vi "Data Retrim.vi"(11 "Data in":dbl[][][](array[numeric])) -> (3 "Data Out":dbl[][][](array[numeric]))   [LabVIEW 2011]
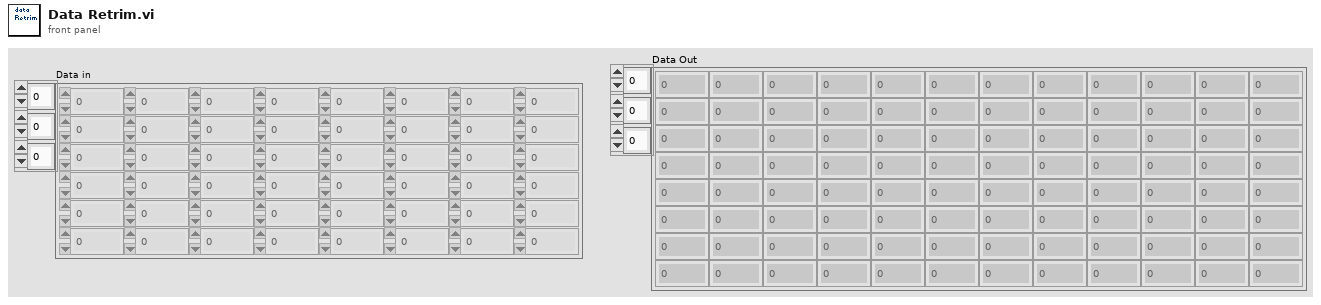
[diagram p1: front panel]
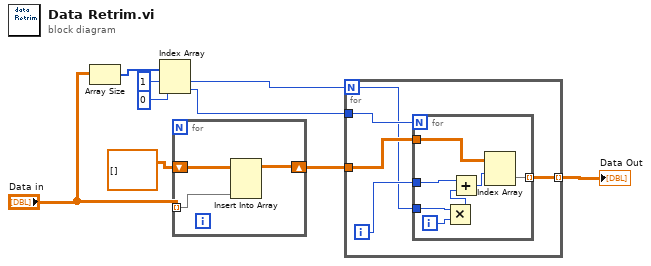
[diagram p0: block diagram]
diagram:
  n1 = Array Size(array="Data in") -> (size(s)=w6:i32[])
  n2 = Index Array(array=w6, index #1=1 ("索引"), index #2=0 ("索引")) -> (element #1=w4:i32, element #2=w2:i32)
  n3 = for {
    tunnel: "Data in" -> [w11] mode=indexing
    shift-right: [w10] -> w8
    shift-left: dbl[][] [] ("Data Out 3") -> [w12]
    n4 = Insert Into Array(array=w12, new element=w11) -> (w10:dbl[][])  [unwired: 2 in]
  }
  n5 = for {
    N: w4 -> [w13]
    tunnel: w8 -> [w17]
    tunnel: w2 -> [w16]
    tunnel: [w14] -> w1 mode=indexing
    i -> [w15]
    n6 = for {
      N: w16 -> [_]
      tunnel: w17 -> [w24]
      tunnel: w15 -> [w22]
      tunnel: [w23] -> w14 mode=indexing
      tunnel: w13 -> [w19]
      i -> [w21]
      n7 = Multiply(x=w19, y=w21) -> (x*y=w20:i32)
      n8 = Add(x=w22, y=w20) -> (x+y=w18:i32)
      n9 = Index Array(array=w24, index (row)=w18) -> (element=w23:dbl[])  [unwired: 1 in]
    }
  }
  "Data Out" <- w1
